vi "Stop Core.vi"(10 "final error code":i32, 11 "CS++Scope in":refnum<class "CS++Scope.lvclass">) -> (3 "CS++Scope out":refnum<class "CS++Scope.lvclass">)   [LabVIEW 2014, in "CS++Scope.lvlib" / "CS++Scope.lvclass"]
doc: "(<B>Filename</B>: Actor Framework.lvlib:Actor.lvclass:Stop Core.vi)\n\nDefines what the actor does before it stops. Use the <B>final error code</B> input to determine whether the actor shut down in response to an error.\n\nBy default, this method does nothing. A descendant class may override it to define behavior, such as shutting down any processes the actor initiated in its override of the Actor Core method."
uses:
  CS++Scope.lvclass
  <vilib>/ActorFramework/Time-Delayed Send Message/Time-Delay Override Options.ctl
  CS++Scope.lvclass/CS++Scope.ctl
  CSPP_Core/Actors/CS++DeviceActor/CS++DeviceActor.lvclass
  CSPP_Core/Classes/CS++ProcessVariables/PVConnection/PVConnection.lvclass
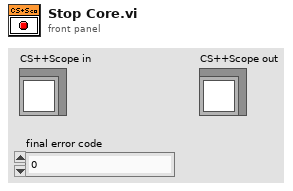
[diagram p1: front panel]
types:
  T1 = typedef "Time-Delay Override Options.ctl" = enum16{"Send next copy now", "Skip next scheduled copy", "Send next copy now and stop all further copies", "Stop all further copies"}
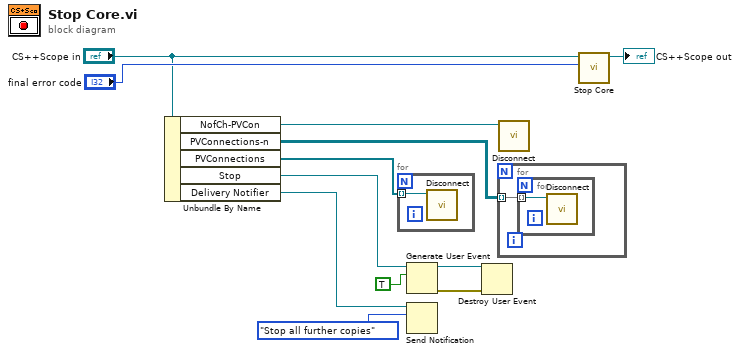
[diagram p0: block diagram]
diagram:
  n1 = Unbundle By Name("CS++Scope in") -> ("NofCh-PVCon"=w8:refnum<class "PVConnection.lvclass">, "PVConnections-n"=w7:refnum<class "PVConnection.lvclass">[][], "PVConnections"=w9:refnum<class "PVConnection.lvclass">[], "Stop"=w4:refnum<user-event>, "Delivery Notifier"=w2:refnum<notifier>)
  n2 = for {
    tunnel: w9 -> [w13] mode=indexing
    n3 = call "Disconnect.vi"("PVConnection in"=w13) -> ()  [unwired: 9 in, 2 out]
  }
  n4 = Generate User Event(user event=w4, event data cluster=TRUE) -> (user event out=w6:refnum<user-event>, error out=w5:errorcluster)  [unwired: 2 in]
  n5 = Send Notification(notification=Time-Delay_Override_Options."Stop all further copies", notifier=w2) -> ()  [unwired: 1 in, 2 out]
  n6 = Destroy User Event(user event=w6, error in=w5) -> ()  [unwired: 1 out]
  n7 = for {
    tunnel: w7 -> [w14] mode=indexing
    n8 = for {
      tunnel: w14 -> [w15] mode=indexing
      n9 = call "Disconnect.vi"("PVConnection in"=w15) -> ()  [unwired: 9 in, 2 out]
    }
  }
  n10 = call "Disconnect.vi"("PVConnection in"=w8) -> ()  [unwired: 9 in, 2 out]
  n11 = call-parent "Stop Core.vi"("final error code"="final error code", "CS++DeviceActor in"="CS++Scope in") -> ("CS++DeviceActor out"=→"CS++Scope out":refnum<class "CS++Scope.lvclass">)  [unwired: 9 in]
